vi "pollScan.vi"(8 "error in (no error)":errorcluster, 10 "Device":i32, 11 "SEDSpectrometer in":refnum<class "SEDSpectrometer.lvclass">) -> (0 "error out":errorcluster, 2 "Output Value":i32, 3 "SEDSpectrometer out":refnum<class "SEDSpectrometer.lvclass">)   [LabVIEW 2016, in "SEDSpectrometer.lvclass"]
uses:
  SEDSpectrometer.lvclass
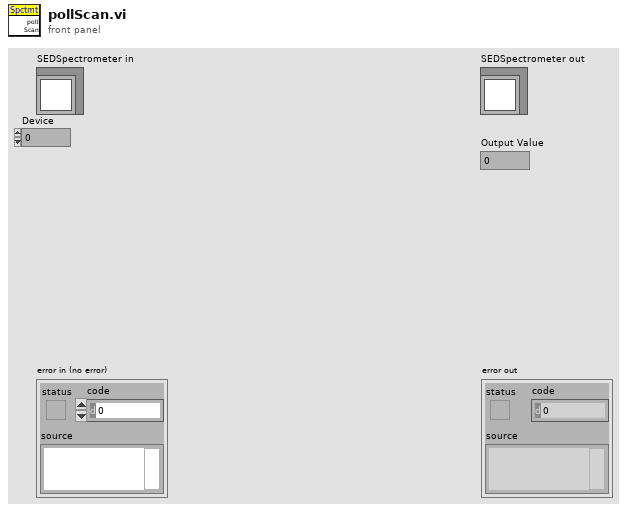
[diagram p1: front panel]
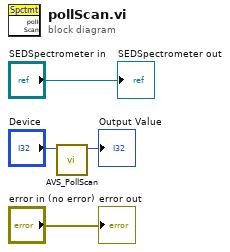
[diagram p0: block diagram]
diagram:
  n1 = call "AVS_PollScan.vi"("a_hDevice"="Device") -> ("Output Value"=→"Output Value":i32)  [unwired: 8 in]
  "error out" <- "error in (no error)"
  "SEDSpectrometer out" <- "SEDSpectrometer in"
